vi "SampleGetIDSingle.vi"() -> ()   [LabVIEW 2009]
panel:
  out "Identification":string
  out "error out":errorcluster
  out "DeviceKey Out":string
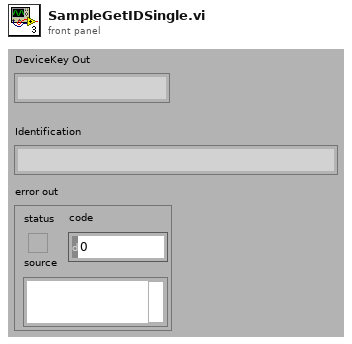
[diagram p1: front panel]
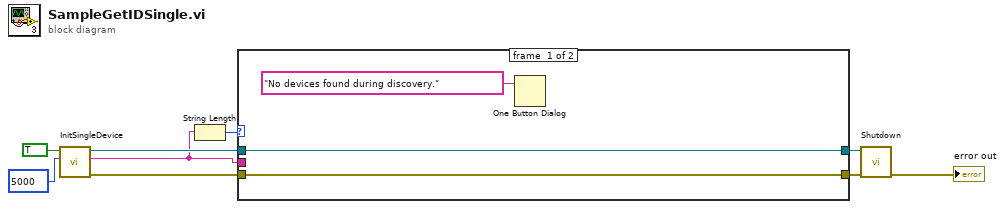
[diagram p0: block diagram]
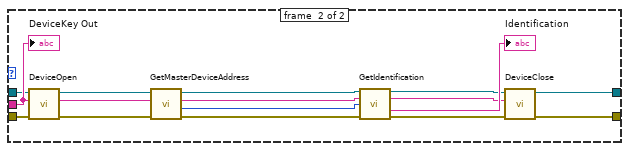
[diagram p2: hidden frame]
diagram:
  n1 = call "InitSingleDevice.vi"("msecDelayForDiscovery"=5000, "logging"=TRUE) -> ("error out"=w2:errorcluster, "DeviceKey Out"=w1:string, "CmdLib Out"=w3:refnum<k24>)  [unwired: 3 in]
  n2 = String Length(string=w1) -> (length=w6:i32)
  n3 = case shown="1, Default" w6 {
    tunnel: [w12 w23] -> w5
    tunnel: [w11 w25] -> w4
    tunnel: w3 -> [w12 w14]
    tunnel: w2 -> [w11 w18]
    tunnel: w1 -> [_ w16]
    frame #0 {
      n4 = One Button Dialog(message="No devices found during discovery.") -> ()  [unwired: 1 in, 1 out]
    }
    frame #1 {
      n5 = call "DeviceOpen.vi"("error in (no error)"=w18, "DeviceKey In"=w16, "CmdLib In"=w14) -> ("error out"=w17:errorcluster, "DeviceKey Out"=w15:string, "CmdLib Out"=w13:refnum<k24>)  [unwired: 2 in]
      n6 = call "GetMasterDeviceAddress.vi"("error in (no error)"=w17, "DeviceKey In"=w15, "CmdLib In"=w13) -> ("error out"=w21:errorcluster, "Device Address"=w27:i32, "DeviceKey Out"=w19:string, "CmdLib Out"=w20:refnum<k24>)  [unwired: 1 in]
      n7 = call "GetIdentification.vi"("CmdLib In"=w20, "DeviceKey In"=w19, "Device Address In"=w27, "error in (no error)"=w21) -> ("CmdLib Out"=w24:refnum<k24>, "DeviceKey Out"=w22:string, "Identification"=→"Identification":string, "error out"=w26:errorcluster)  [unwired: 7 in, 1 out]
      n8 = call "DeviceClose.vi"("error in (no error)"=w26, "DeviceKey In"=w22, "CmdLib In"=w24) -> ("error out"=w25:errorcluster, "CmdLib Out"=w23:refnum<k24>)  [unwired: 2 in, 1 out]
      "DeviceKey Out" <- w16
    }
  }
  n9 = call "Shutdown.vi"("error in (no error)"=w4, "CmdLib In"=w5) -> ("error out"=→"error out":errorcluster)  [unwired: 4 in, 1 out]
